vi "Move String Block.vi"(0 "src buffer in":u8[](array[numeric]), 1 "dst buffer in":u8[](array[numeric]), 2 "src buffer offset":u64 format="%d bytes", 3 "dst buffer offset":u64 format="%d bytes", 4 "channel count":u64, 5 "error in (no error)":errorcluster, 6 "dst data type":T1, 8 "src data type":T1, 10 "dst byte order":T2(ring), 12 "src byte order":T2(ring)) -> (14 "src buffer out":u8[](array[numeric]), 15 "dst buffer out":u8[](array[numeric]), 19 "error out":errorcluster)   [LabVIEW 2017, in "DSF Core.lvlib" / "Default Buffer Converter.lvclass"]
uses:
  Default Buffer Converter.lvclass
  Typedefs/DSF Data Type.ctl
  Classes/Framework/Framework.lvclass
  Classes/Buffer Converter/Buffer Converter.lvclass
  DSF Core.lvlib
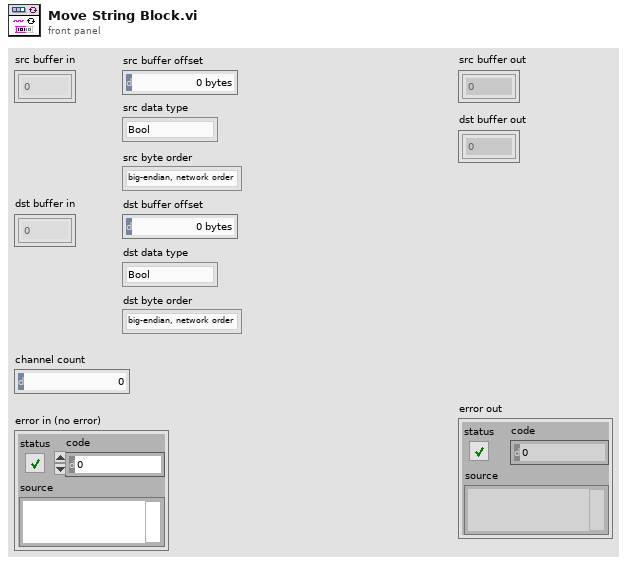
[diagram p1: front panel]
types:
  T1 = typedef "DSF Core.lvlib/DSF Data Type.ctl" = enum8{"Bool", "SGL", "DBL", "I8", "I16", "I32", "I64", "U8", "U16", "U32", "U64"}
  T2 = enum16{"big-endian, network order", "native, host order", "little-endian"}
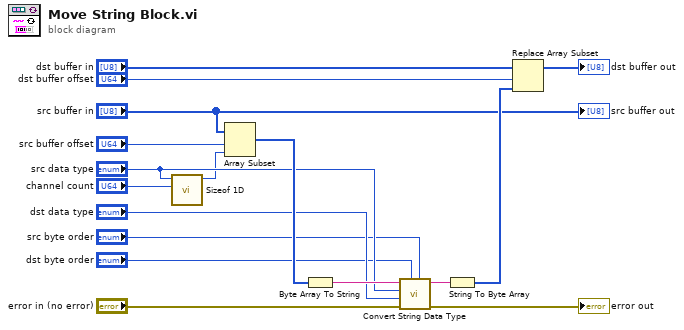
[diagram p0: block diagram]
diagram:
  n1 = call "Sizeof 1D.vi"("count"="channel count", "data type"="src data type") -> ("size in bytes"=w3:u64)  [unwired: 9 in]
  n2 = Array Subset(array="src buffer in", index="src buffer offset", length=w3) -> (w10:u8[])
  n3 = Byte Array To String(unsigned byte array=w10) -> (string=w6:string)
  n4 = call "Convert String Data Type.vi"("src byte order"="src byte order", "dst byte order"="dst byte order", "error in (no error)"="error in (no error)", "dst data type"="dst data type", "src data type"="src data type", "src data in"=w6) -> ("error out"=→"error out":errorcluster, "dst data out"=w7:string)  [unwired: 4 in]
  n5 = String To Byte Array(string=w7) -> (unsigned byte array=w14:u8[])
  n6 = Replace Array Subset(array="dst buffer in", new element=w14, index="dst buffer offset") -> (→"dst buffer out":u8[])
  "src buffer out" <- "src buffer in"
